vi "test_RemoteDCPowerSession_CallInitializeMeasurementLinkSessionWithAttachBehavior_RemoteSessionAttached.vi"(8 "error in":errorcluster) -> (0 "error out":errorcluster, 2 "result":string, 3 "pass":bool)   [LabVIEW 2020, in "MeasurementServerTests.lvlib"]
uses:
  MeasurementServerTests.lvlib
  Runtime/MeasurementLink niDCPower/Session Factory/Session Factory.lvclass
  Runtime/MeasurementLink Instrument/ISession Factory/Initialize and Close Session Behavior.ctl
  Runtime/MeasurementLink Instrument/ISession Factory/ISession Factory.lvclass
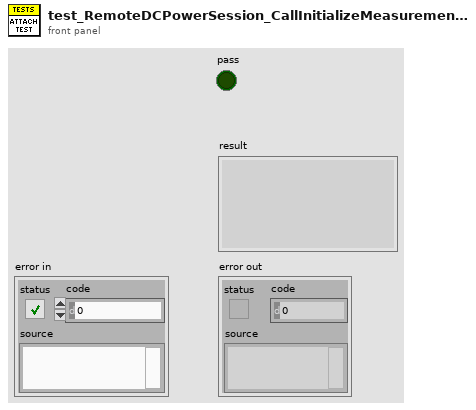
[diagram p1: front panel]
types:
  T1 = typedef "MeasurementLink Instrument.lvlib/ISession Factory.lvclass/Remote Connection Options.ctl" = cluster{"session name":string, "address":string, "port":u32}
  T2 = typedef "MeasurementLink Instrument.lvlib/ISession Factory.lvclass/Initialize and Close Session Behavior.ctl" = enum16{"Initialize and Close", "Attach and Detach", "Initialize and Detach", "Attach and Close"}
  T3 = typedef "MeasurementLink Instrument.lvlib/ISession Factory.lvclass/Session Initialization Parameters.ctl" = cluster{"resource name":string, "session name":string}
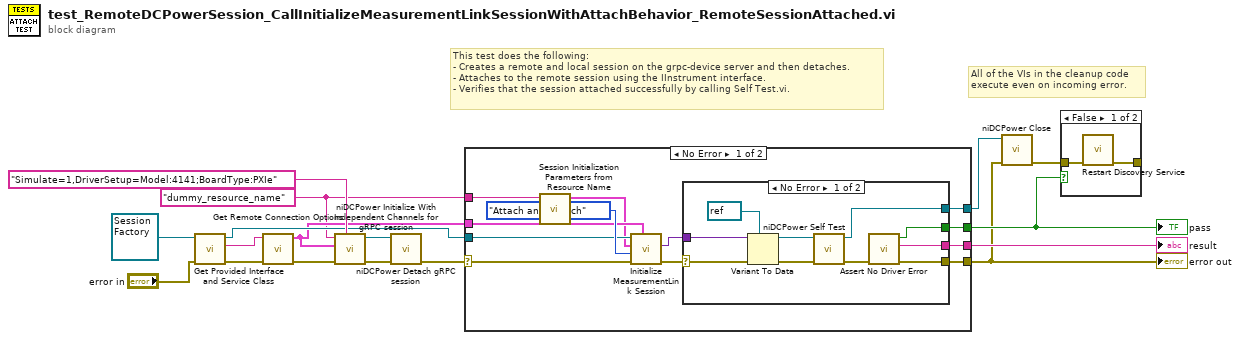
[diagram p0: block diagram]
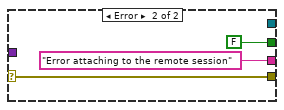
[diagram p2: hidden frame]
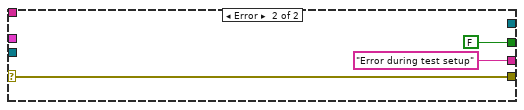
[diagram p3: hidden frame]
diagram:
  w1 = "dummy_resource_name" ("resource name")
  # "All of the VIs in the cleanup code\nexecute even on incoming error."
  # "This test does the following:\n- Creates a remote and local session on the grpc-device server and then detaches.\n- Attaches to the remote session using the IInstrument interface.\n- Verifies that the session attached successfully by calling Self Test.vi."
  n1 = call-dynamic "Get Provided Interface and Service Class.vi"("error in"="error in", "session factory in"=refnum<class "Session Factory.lvclass"> refnum ("MeasurementLink niDCPower.lvlib:Instrument.lvclass")) -> ("error out"=w9:errorcluster, "provided interface"=w8:string, "session factory out"=w6:refnum<class "Session Factory.lvclass">)  [unwired: 6 in, 1 out]
  n2 = call "Get Remote Connection Options.vi"("error in"=w9, "provided interface"=w8) -> ("error out"=w11:errorcluster, "remote connection options"=w2:T1)  [unwired: 8 in]
  n3 = call <instrlib>:"niDCPower Initialize With Independent Channels for gRPC session.vi"("option string"="Simulate=1,DriverSetup=Model:4141;BoardType:PXIe", "error in (no error)"=w11, "gRPC options"=w2, "resource name"=w1) -> ("error out"=w5:errorcluster, "instrument handle out"=w3:refnum<k15>)  [unwired: 6 in]
  n4 = call <instrlib>:"niDCPower Detach gRPC session.vi"("error in (no error)"=w5, "instrument handle"=w3) -> ("error out"=w4:errorcluster)  [unwired: 9 in]
  n5 = case shown="No Error" w4 {
    selector: w4 -> [w23 w43]
    tunnel: [w28 w43] -> w13
    tunnel: [w29 FALSE] -> w14
    tunnel: [w27 "Error during test setup" ("f")] -> w17
    tunnel: w6 -> [w22 _]
    tunnel: [w21 _] -> w16
    tunnel: w2 -> [w20 _]
    tunnel: w1 -> [w19 _]
    frame No Error {
      n6 = call "Session Initialization Parameters from Resource Name.vi"("resource name"=w19) -> ("session initialization parameters"=w18:T3)  [unwired: 10 in]
      n7 = call-dynamic "Initialize MeasurementLink Session.vi"("remote connection options"=w20, "error in"=w23, "initialize and close session behavior"=Initialize_and_Close_Session_Behavior."Attach and Detach", "session initialization parameters"=w18, "session factory in"=w22) -> ("error out"=w25:errorcluster, "session out"=w26:variant)  [unwired: 4 in, 1 out]
      n8 = case shown="No Error" w25 {
        selector: w25 -> [w38 w41]
        tunnel: [w32 FALSE] -> w29
        tunnel: [w30 w41] -> w28
        tunnel: [w31 "Error attaching to the remote session"] -> w27
        tunnel: w26 -> [w39 _]
        tunnel: [w34 _] -> w21
        frame No Error {
          n9 = Variant To Data(error in=w38, type=refnum<k15> refnum ("instrument handle"), Variant=w39) -> (data=w35:refnum<k15>, error out=w36:errorcluster)
          n10 = call <instrlib>:"niDCPower Self Test.vi"("error in (no error)"=w36, "instrument handle"=w35) -> ("error out"=w33:errorcluster, "instrument handle out"=w34:refnum<k15>)  [unwired: 6 in, 2 out]
          n11 = call "Assert No Driver Error.vi"("error in"=w33) -> ("error out"=w30:errorcluster, "result"=w31:string, "pass?"=w32:bool)  [unwired: 8 in]
        }
        frame Error {
        }
      }
    }
    frame Error {
    }
  }
  "error out" <- w13
  "pass" <- w14
  "result" <- w17
  n12 = call <instrlib>:"niDCPower Close.vi"("error in (no error)"=w13, "instrument handle"=w16) -> ("error out"=w15:errorcluster)  [unwired: 9 in]
  n13 = case shown="False" w14 {
    tunnel: w15 -> [w47 _]
    tunnel: [w46 _] -> _
    frame False {
      n14 = call "Restart Discovery Service.vi"("error in"=w47) -> ("error out"=w46:errorcluster)  [unwired: 10 in]
    }
    frame True {
    }
  }
